vi "Recieve Timer Tick.vi"(8 "error in (no error)":errorcluster, 10 "Time Stamp Control":timestamp, 11 "Common Measurements in":refnum<class "Common Measurements.lvclass">) -> (0 "error out":errorcluster, 3 "Common Measurements out":refnum<class "Common Measurements.lvclass">)   [LabVIEW 2015, in "Common Measurements.lvclass"]
uses:
  Common Measurements.lvclass
  Mag Lab Measure Base/Mag Lab Measure Base.lvclass/Mag Lab Measure Base.ctl
  Common Measurements Interface Messages/Update time Msg/Update time Msg.lvclass/Update time Msg.ctl
  <vilib>/ActorFramework/Message Enqueuer/Message Enqueuer.lvclass/Message Enqueuer.ctl
  <vilib>/ActorFramework/Message Enqueuer/Enqueue.vi
  <vilib>/ActorFramework/Message Priority Queue/Priority Enqueue.vi
  Mag Lab Measure Controller/Mag Lab Measure Controller.lvclass
  <vilib>/ActorFramework/Message Enqueuer/Message Enqueuer.lvclass
  Common Measurements Interface Messages/Update time Msg/Update time Msg.lvclass
  Mag Lab Measure Base/Mag Lab Measure Base.lvclass
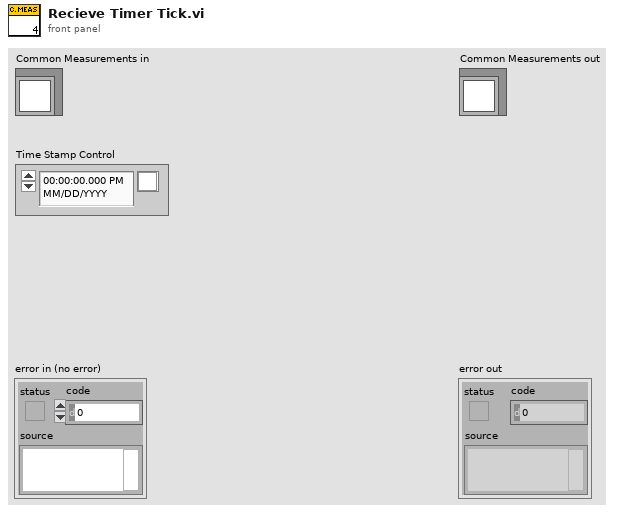
[diagram p1: front panel]
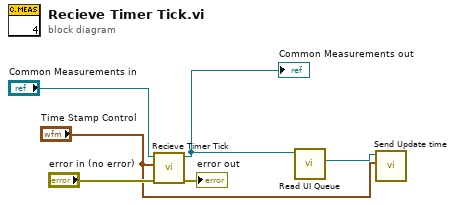
[diagram p0: block diagram]
diagram:
  n1 = call-parent "Recieve Timer Tick.vi"("error in (no error)"="error in (no error)", "Time Stamp Control"="Time Stamp Control", "Mag Lab Measure Controller in"="Common Measurements in") -> ("error out"=→"error out":errorcluster, "Mag Lab Measure Controller out"=w3:refnum<class "Common Measurements.lvclass">)  [unwired: 7 in]
  "Common Measurements out" <- w3
  n2 = call "Read UI Queue.vi"("Mag Lab Measure Base in"=w3) -> ("Actor Framework.lvlib:Message Enqueuer"=w2:refnum<class "Message Enqueuer.lvclass">)  [unwired: 8 in, 2 out]
  n3 = call "Send Update time.vi"("Time Stamp Control"="Time Stamp Control", "Message Enqueuer"=w2) -> ()  [unwired: 8 in, 2 out]
